vi "WPI_SerialPortReset.vi"(8 "error in (no error)":errorcluster, 11 "SerialPortRef":T1) -> (0 "error out":errorcluster, 3 "SerialPortRef":T1)   [LabVIEW 2017]
doc: "Clears the input and output buffers of the serial device you specify.\n\nThis software is licensed. Open the labview\\readme\\WPI Robotics Library Open Source License.txt file for more information."
uses:
  <vilib>/Rock Robotics/WPI/SerialPort/WPI_SerialPortRef.ctl
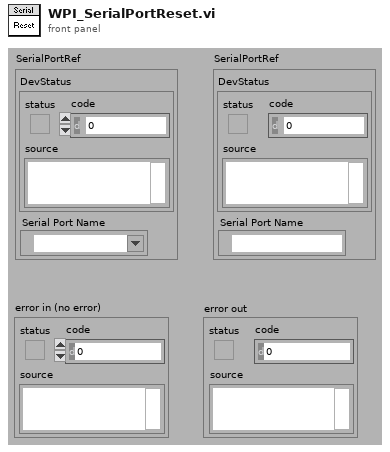
[diagram p1: front panel]
types:
  T1 = typedef "WPI_SerialPortRef.ctl" = cluster{"DevStatus":errorcluster, "Serial Port Name":refnum<visa-resource-name>}
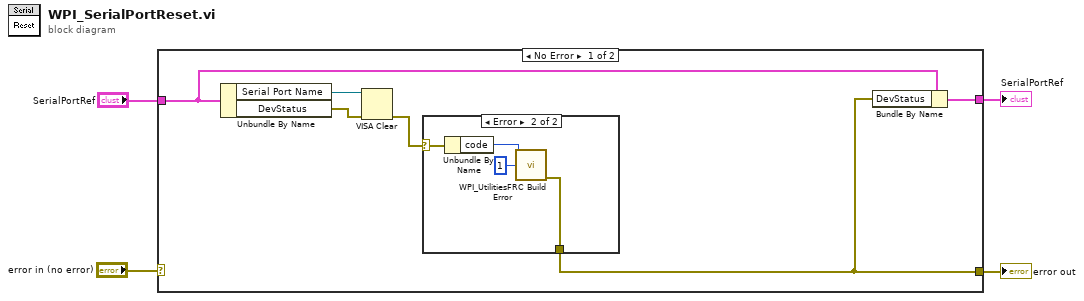
[diagram p0: block diagram]
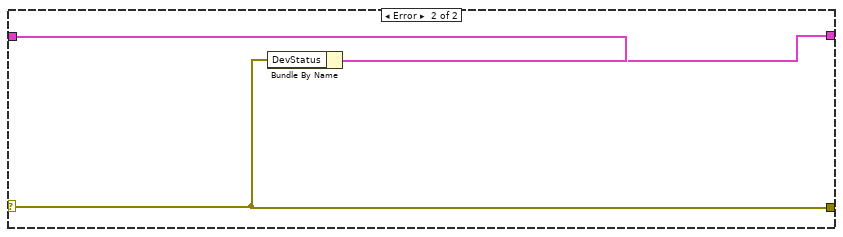
[diagram p3: hidden frame]
diagram:
  n1 = case shown="No Error" "error in (no error)" {
    selector: "error in (no error)" -> [_ w16]
    tunnel: "SerialPortRef" -> [w10 w18]
    tunnel: [w9 w17] -> w3
    tunnel: [w5 w16] -> w1
    frame No Error {
      n2 = Unbundle By Name(w10) -> ("Serial Port Name"=w8:refnum<visa-resource-name>, "DevStatus"=w7:errorcluster)
      n3 = VISA Clear(VISA resource name=w8, error in (no error)=w7) -> (error out=w6:errorcluster)  [unwired: 1 out]
      n4 = case shown="Error" w6 {
        selector: w6 -> [w11 w13]
        tunnel: [w11 w12] -> w5
        frame No Error {
        }
        frame Error {
          n5 = Unbundle By Name(w13) -> ("code"=w15:i32)
          n6 = call <vilib>:"WPI_UtilitiesFRC Build Error.vi"("error code"=w15, "chain levels to remove (1)"=1) -> ("error out"=w12:errorcluster)  [unwired: 3 in, 10 out]
        }
      }
      n7 = Bundle By Name(cluster=w10, "DevStatus"=w5) -> (w9:T1)
    }
    frame Error {
      n8 = Bundle By Name(cluster=w18, "DevStatus"=w16) -> (w17:T1)
    }
  }
  "error out" <- w1
  "SerialPortRef" <- w3
